vi "WC Number of Waveform Samples CDBL.vi"(8 "error in (no error)":errorcluster, 11 "Waveform In":cluster{"t0":dbl, "dt":dbl, "Y":cdb[]} {"Y" format="%.3p"; "dt" format="%.6p"; "t0" format="%.6p"}) -> (0 "error out":errorcluster, 2 "number of samples":i32, 3 "Waveform Out":cluster{"t0":dbl, "dt":dbl, "Y":cdb[]} {"Y" format="%.3p"; "dt" format="%.6p"; "t0" format="%.6p"})   [LabVIEW 2018]
doc: "Returns the number of data elements in the waveform. You must manually select the polymorphic instance you want to use."
panel:
  in  "Waveform Error":cluster{"t0":dbl, "dt":dbl, "Y":cdb[]} {"Y" format="%.3p"; "dt" format="%.6p"; "t0" format="%.6p"}
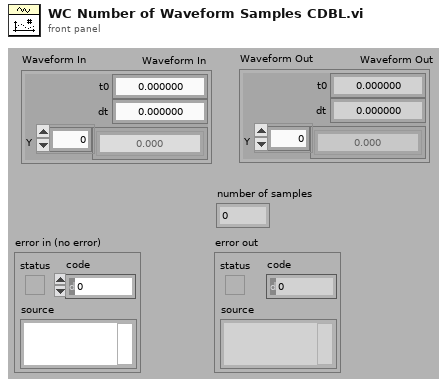
[diagram p1: front panel]
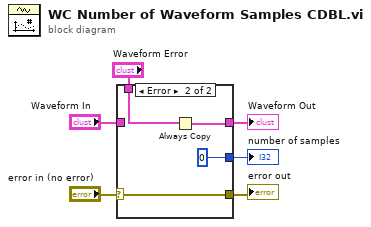
[diagram p0: block diagram]
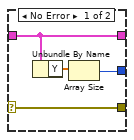
[diagram p2: hidden frame]
diagram:
  n1 = case shown="Error" "error in (no error)" {
    selector: "error in (no error)" -> [w9 w13]
    tunnel: "Waveform In" -> [w8 _]
    tunnel: [w8 w12] -> w5
    tunnel: [w10 0] -> w6
    tunnel: "Waveform Error" -> [_ w11]
    tunnel: [w9 w13] -> w2
    frame No Error {
      n2 = Unbundle By Name(w8) -> ("Y"=w7:cdb[])
      n3 = Array Size(array=w7) -> (size(s)=w10:i32)
    }
    frame Error {
      # "Incoming Error"
      n4 = Always Copy(1:w11) -> (0:w12:cluster{"t0":dbl, "dt":dbl, "Y":cdb[]})
    }
  }
  "number of samples" <- w6
  "Waveform Out" <- w5
  "error out" <- w2
